vi "event_functional_stop.vi"(6 "functional":refnum<user-event>, 8 "error in (no error)":errorcluster) -> (0 "error out":errorcluster)   [LabVIEW 2015, in "functional.lvlib"]
uses:
  functional.lvlib
  _controls/event_functional.ctl
  _controls/event_functional_command.ctl
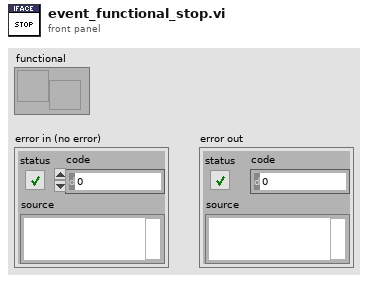
[diagram p1: front panel]
types:
  T1 = typedef "functional.lvlib/event_functional.ctl" = cluster{"command":T2, "data":variant}
  T2 = typedef "functional.lvlib/event_functional_command.ctl" = enum16{"<command_functional>", "--high-level", "stop", "update_hmi_references", "load_interface", "--functional", "do_it", "<null>"}
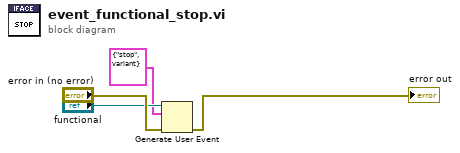
[diagram p0: block diagram]
diagram:
  n1 = Generate User Event(user event="functional", event data cluster=T1 {"command"=enum."stop", "data"=variant} ("event data"), error in="error in (no error)") -> (error out=→"error out":errorcluster)  [unwired: 1 in, 1 out]
